vi "New Client from Socket.vi"(8 "error in (no error)":errorcluster, 10 "WebSocket URL":string, 11 "Socket in":refnum<class "Socket.lvclass">) -> (0 "error out":errorcluster, 3 "WebSocket Client out":refnum<class "WebSocket Client.lvclass">)   [LabVIEW 2013, in "WebSockets.lvlib" / "WebSocket Client.lvclass"]
doc: "Creates a new WebSockets Client connection from an existing Socket object."
uses:
  WebSocket Client.lvclass
  Sockets/Socket/Socket.lvclass
  WebSocket/WebSocket.lvclass/WebSocket.ctl
  WebSocket Client.lvclass/WebSocket Client.ctl
  WebSocket/Write Socket.vi
  Write URL.vi
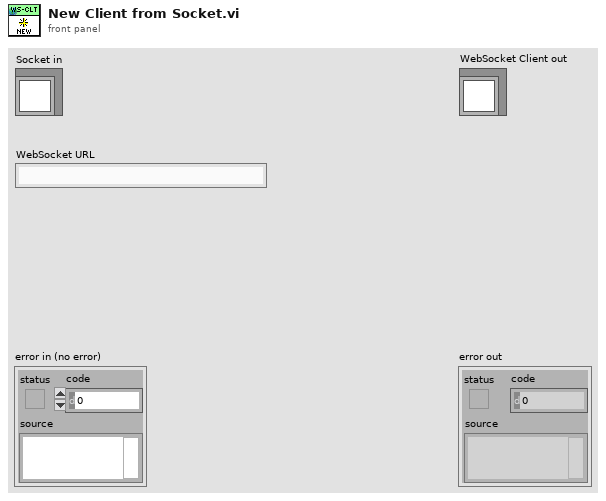
[diagram p1: front panel]
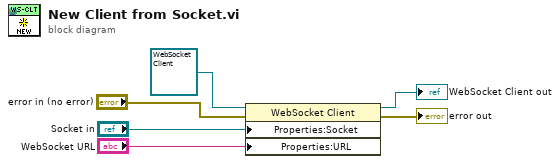
[diagram p0: block diagram]
diagram:
  n1 = property class="WebSocket Client"(reference=refnum<class "WebSocket Client.lvclass"> refnum ("WebSocket Client in"), error in="error in (no error)", "Properties:Socket"="Socket in", "Properties:URL"="WebSocket URL") -> (reference out=→"WebSocket Client out":refnum<class "WebSocket Client.lvclass">, error out=→"error out":errorcluster)
